vi "AddClassChildrenToClassMetadata.vi"(6 "Children[]":refnum<vi>[](array[refnum]), 8 "error in":errorcluster, 11 "ClassMetadata instance":refnum<data-value>) -> (0 "error out":errorcluster, 3 "ClassMetadata instance out":refnum<data-value>)   [LabVIEW 2017]
uses:
  Helpers/DirectoryMetadata/DirectoryMetadata.lvclass
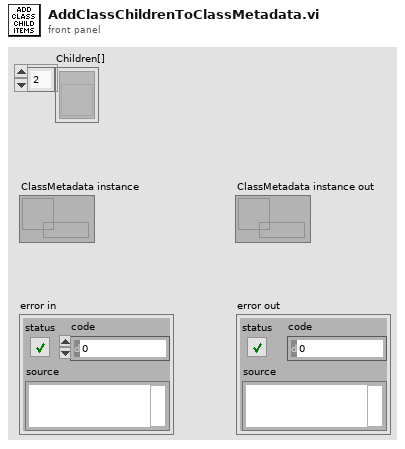
[diagram p1: front panel]
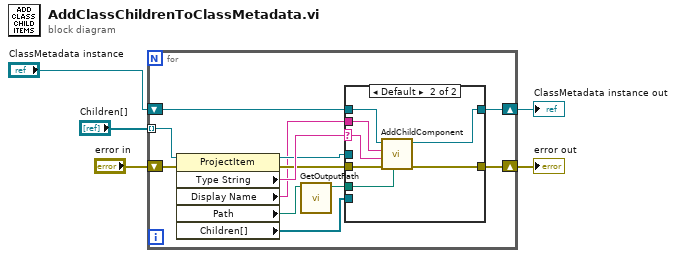
[diagram p0: block diagram]
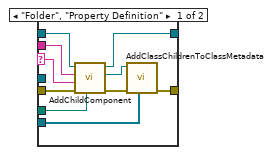
[diagram p2: hidden frame]
diagram:
  n1 = for {
    tunnel: "Children[]" -> [w17] mode=indexing
    shift-right: [w14] -> w3
    shift-left: "error in" -> [w13]
    shift-right: [w10] -> w1
    shift-left: "ClassMetadata instance" -> [w11]
    n2 = property class="ProjectItem"(reference=w17, error in=w13) -> (reference out=w15:refnum<vi>, error out=w12:errorcluster, "Type String"=w16:string, "Display Name"=w7:string, "Path"=w9:path, "Children[]"=w6:refnum<vi>[])
    n3 = call "GetOutputPath.vi"("Path"=w9) -> ("Output Path"=w8:path)  [unwired: 10 in]
    n4 = case shown="Default" w16 {
      selector: w16 -> [w26 w33]
      tunnel: w15 -> [_ _]
      tunnel: w12 -> [w23 w31]
      tunnel: [w24 w30] -> w14
      tunnel: w11 -> [w27 w34]
      tunnel: [w25 w32] -> w10
      tunnel: w8 -> [w19 w29]
      tunnel: w7 -> [w20 w28]
      tunnel: w6 -> [w18 _]
      frame "Folder", "Property Definition" {
        n5 = call "AddChildComponent.vi"("Path"=w19, "error in (no error)"=w23, "Type"=w26, "ID"=w20, "head in"=w27) -> ("error out"=w22:errorcluster, "child ref"=w21:refnum<data-value>, "head out"=w25:refnum<data-value>)  [unwired: 4 in]
        n6 = call "AddClassChildrenToClassMetadata.vi"("Children[]"=w18, "error in"=w22, "ClassMetadata instance"=w21) -> ("error out"=w24:errorcluster)  [unwired: 7 in, 1 out]
      }
      frame Default {
        n7 = call "AddChildComponent.vi"("Path"=w29, "error in (no error)"=w31, "Type"=w33, "ID"=w28, "head in"=w34) -> ("error out"=w30:errorcluster, "head out"=w32:refnum<data-value>)  [unwired: 4 in, 1 out]
      }
    }
  }
  "error out" <- w3
  "ClassMetadata instance out" <- w1
